vi "Constants.vi"() -> ()   [LabVIEW 2020, in "gRPC Data Server Shared.lvlib"]
doc: "Use this Global VI to access the GUIDs assigned to the page resources of the Custom Device."
uses:
  gRPC Data Server Shared.lvlib
panel:
  in  "Tab Control":enum32{"GUIDs", "Constants", "Properties"}(tab)
  in  "Data Server":string="50607266-7804-459d-9f58-da99f817b781"
  in  "gRPC Data Server":string="3d66a51a-0196-4a83-8de6-7f3c7163e92c"
  in  "Server.Channel Name":string="Server.Channel Name"
  in  "Server.Initial Value":string="Server.Initial Value"
  in  "Server.Cert File":string="Server.Cert File"
  in  "Server.Key File":string="Server.Key File"
  in  "Server.Async?":string="Server.Async?"
  in  "Server.Address":string="Server.Address"
  in  "Compiled.Settings":string="Compiled.Settings"
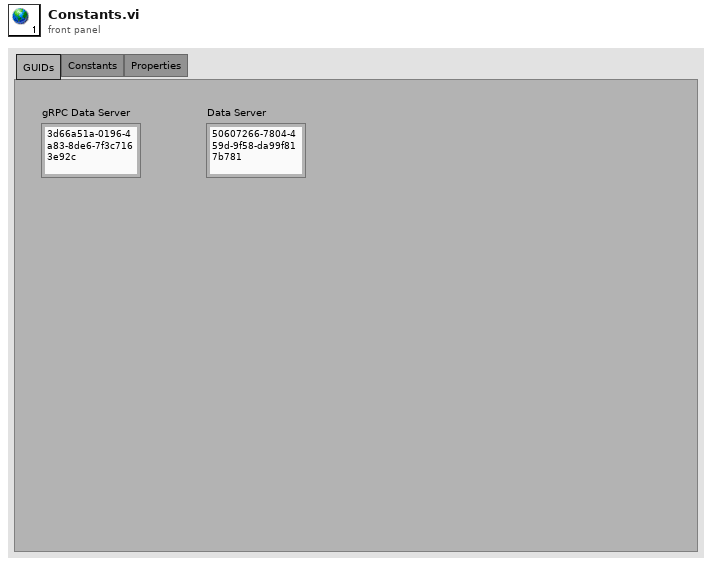
[diagram p1: front panel]
diagram:
